vi "onDecodeHeaderString.vi"(8 "error in (no error)":errorcluster, 10 "http-header (unparsed)":string, 11 "httpHeaders":refnum<class "httpHeaders.lvclass">) -> (0 "error out":errorcluster, 2 "headers":cluster{"header":string, "value":string}[](array[cluster]))   [LabVIEW 2020, in "httpClient.lvlib" / "httpHeaders.lvclass"]
uses:
  httpHeaders.lvclass
  httpHeaders.lvclass/httpHeaders.ctl
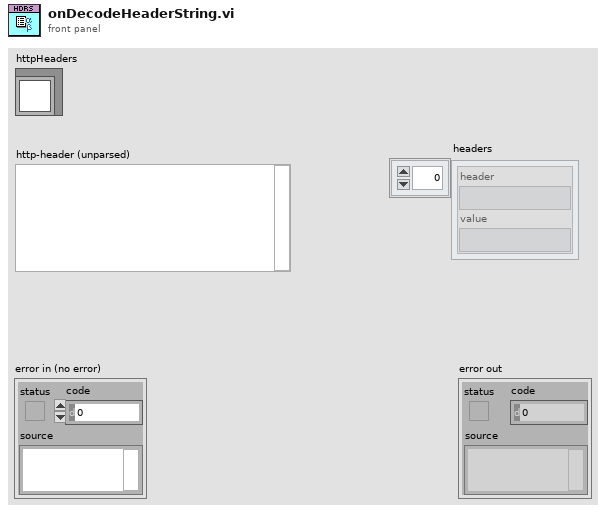
[diagram p1: front panel]
types:
  T1 = cluster{"trimmed string":string, "trimmed string":string}
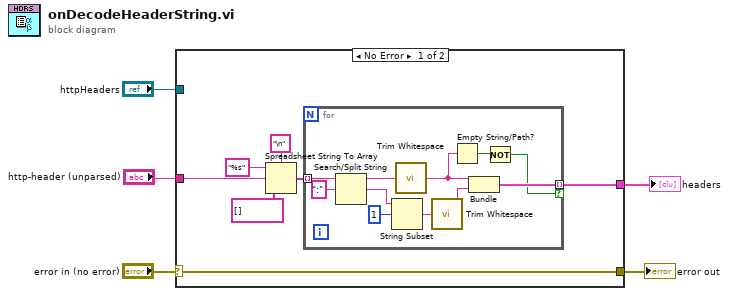
[diagram p0: block diagram]
diagram:
  n1 = case shown="No Error" "error in (no error)" {
    selector: "error in (no error)" -> [w12 w24]
    tunnel: [w12 w24] -> w4
    tunnel: [w7 _] -> w3
    tunnel: "http-header (unparsed)" -> [w6 _]
    tunnel: "httpHeaders" -> [_ _]
    frame No Error {
      n2 = Spreadsheet String To Array(delimiter (Tab)="\n", format string="%s", spreadsheet string=w6, array type (2D Dbl)=string[] []) -> (array=w8:string[])
      n3 = for {
        tunnel: w8 -> [w23] mode=indexing
        tunnel: [w20] -> w7 mode=indexing if=w15
        n4 = Search/Split String(string=w23, search string/char (-)=":") -> (substring before match=w14:string, match + rest of string=w19:string)  [unwired: 1 in, 1 out]
        n5 = String Subset(string=w19, offset (0)=1) -> (substring=w17:string)  [unwired: 1 in]
        n6 = call <vilib>:"Trim Whitespace.vi"("string"=w14) -> ("trimmed string"=w13:string)  [unwired: 1 in]
        n7 = call <vilib>:"Trim Whitespace.vi"("string"=w17) -> ("trimmed string"=w21:string)  [unwired: 1 in]
        n8 = Empty String/Path?(string/path=w13) -> (empty?=w16:bool)
        n9 = Bundle("trimmed string"=w13, "trimmed string"=w21) -> (w20:T1)  [unwired: 1 in]
        n10 = Not(x=w16) -> (.not. x?=w15:bool)
      }
    }
    frame Error {
    }
  }
  "error out" <- w4
  "headers" <- w3
